vi "Pre Launch Init.vi"(11 "PublishingModel In":refnum<class "PublishingModel.lvclass">) -> (0 "error out":errorcluster, 3 "PublishingModel Out":refnum<class "PublishingModel.lvclass">)   [LabVIEW 2017, in "TestPubSubRouting.lvlib" / "PublishingModel.lvclass"]
doc: "(<B>Filename</B>: Actor Framework.lvlib:Actor.lvclass:Pre Launch Init.vi)\n\nDefines behavior that occurs after the Launch Nested Actor method is invoked but before the actor's Actor Core method begins running.\n\nBy default, this method does nothing. A descendant class may override it to define behavior."
uses:
  PublishingModel.lvclass
  gpm_packages/@cs/mva-core/Source/IModel/IModel/IModel.lvclass
  C:/Git/mva-framework/Source/Framework/IModel/IModel/IModel.lvclass
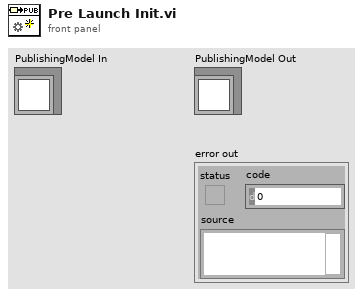
[diagram p1: front panel]
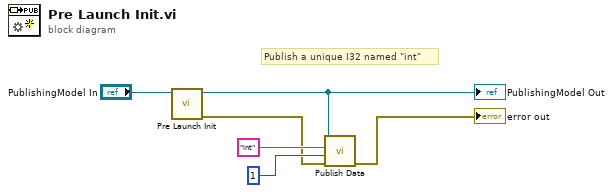
[diagram p0: block diagram]
diagram:
  # "Publish a unique I32 named \"int\""
  n1 = call-parent "Pre Launch Init.vi"("IModel in"="PublishingModel In") -> ("error out"=w2:errorcluster, "IModel out"=w5:refnum<class "PublishingModel.lvclass">)  [unwired: 9 in]
  "PublishingModel Out" <- w5
  n2 = call "Publish Data.vi"("error in (no error)"=w2, "Data to Publish"=1, "Datum Name"="int", "IModel in"=w5) -> ("error out"=→"error out":errorcluster)  [unwired: 6 in, 1 out]
